vi "file handling_0.vi"() -> ()   [LabVIEW 2015]
panel:
  in  "stop 2":bool
  in  "stop":bool
  in  "Tab Control":enum32{"Write to text", "Read from text"}(tab)
  in  "file path (use dialog)":path
  in  "text":string
  in  "file path (use dialog) 2":path
  out "text 2":string
  # "Pardeep Kumar"
  # "Pardeep Kumar"
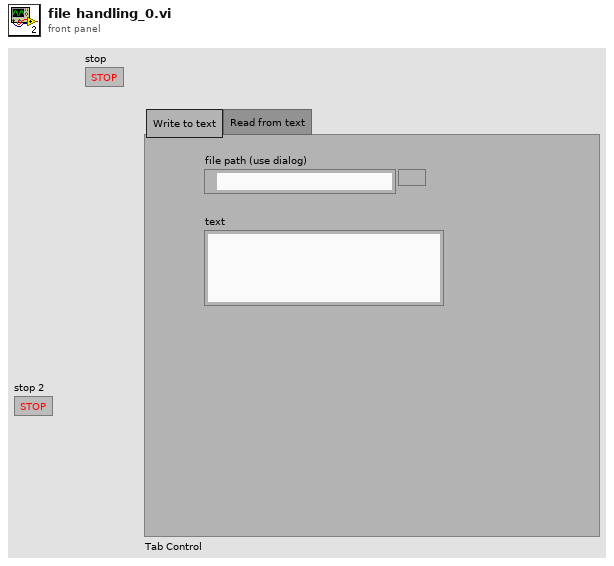
[diagram p1: front panel]
types:
  T1 = enum16{"open", "replace", "create", "open or create", "replace or create", "replace or create with confirmation"}
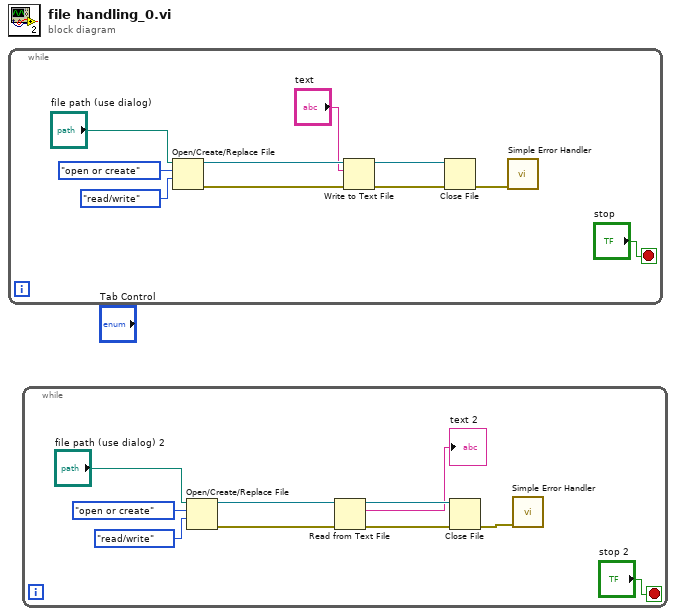
[diagram p0: block diagram]
diagram:
  n1 = while {
    stop <- "stop" stop-if-true
    n2 = Open/Create/Replace File(file path (use dialog)="file path (use dialog)", operation (0:open)=T1."open or create", access (0:read/write)=enum16{"read/write", "read-only", "write-only"}."read/write") -> (refnum out=w10:refnum<file>, error out=w7:errorcluster)  [unwired: 3 in, 1 out]
    n3 = Write to Text File(file (use dialog)=w10, text="text", error in=w7) -> (refnum out=w9:refnum<file>, error out=w8:errorcluster)  [unwired: 1 in, 1 out]
    n4 = Close File(refnum=w9, error in=w8) -> (error out=w2:errorcluster)  [unwired: 1 out]
    n5 = call <vilib>:"Simple Error Handler.vi"("error in (no error)"=w2) -> ()  [unwired: 4 in, 5 out]
  }
  n6 = while {
    stop <- "stop 2" stop-if-true
    n7 = Open/Create/Replace File(file path (use dialog)="file path (use dialog) 2", operation (0:open)=T1."open or create", access (0:read/write)=enum16{"read/write", "read-only", "write-only"}."read/write") -> (refnum out=w20:refnum<file>, error out=w17:errorcluster)  [unwired: 3 in, 1 out]
    n8 = Read from Text File(file (use dialog)=w20, error in=w17) -> (refnum out=w19:refnum<file>, text=→"text 2":string, error out=w18:errorcluster)  [unwired: 2 in, 1 out]
    n9 = Close File(refnum=w19, error in=w18) -> (error out=w13:errorcluster)  [unwired: 1 out]
    n10 = call <vilib>:"Simple Error Handler.vi"("error in (no error)"=w13) -> ()  [unwired: 4 in, 5 out]
  }
